vi "Set_Parameter_Instrument (Json).vi"(8 "error in (no error)":errorcluster caption="entrée d'erreur (pas d'erreur)", 10 "Parameter (Json)":string, 11 "Show_Information en entrée":refnum<class "Wait_OpenFixture.lvclass">) -> (0 "error out":errorcluster caption="sortie d'erreur", 3 "Show_Information en sortie":refnum<class "Wait_OpenFixture.lvclass">)   [LabVIEW 2020, in "Library Test.lvlib" / "Wait_OpenFixture.lvclass"]
uses:
  Wait_OpenFixture.lvclass
  C:/Users/ngarcin/OneDrive - Altyor/Standard TB/Class/Test/Test (Default)/Test (Default).lvclass
  Commun VI/TypeDef/Commande DIO/Parameter DIO.ctl
  DIO/Class DIO (Default)/Class DIO (Default).lvclass
  Wait_OpenFixture.lvclass/Wait_OpenFixture.ctl
  JSON API/JSON Value/Set from JSON string.vi
  JSON API/Variant JSON/Variant to JSON.vi
  JSON API/JSON Value/Get Item by name array.vi
  Test_Without_Instr/Test_Without_Inst.lvclass
  Instrument/Instrument (Default)/Class Instrument (Default).lvclass
  JSON API/JSON Value/JSON Value.lvclass
  JSON API/Variant JSON/Variant JSON.lvlib
  JSON API/Get Polymorphic/JSON GetSet.lvlib
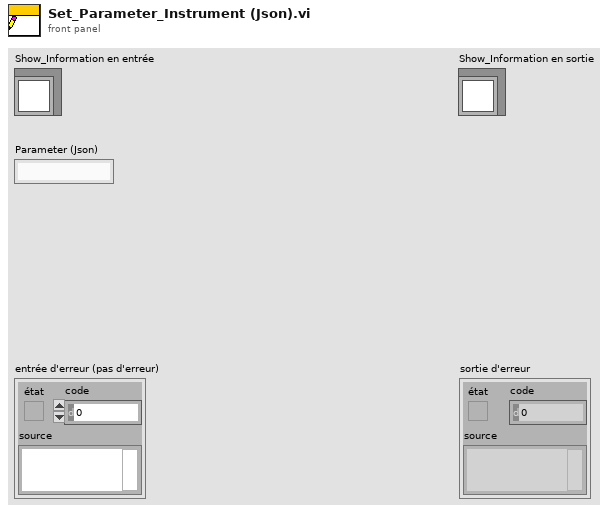
[diagram p1: front panel]
types:
  T1 = cluster{"Information_Operator":string, "Ok_Button_Visible":bool, "Path_Picture":path, "Timeout (ms)":u64, "Function":enum16{"Write", "Read"}, "Line":u8, "Port":u8}
  T2 = typedef "Parameter DIO.ctl" = cluster{"Device_Com_Port":string, "Port":u8, "Line":u8, "Function":enum16{"Write", "Read"}, "Class DIO":refnum<class "Class DIO (Default).lvclass">}
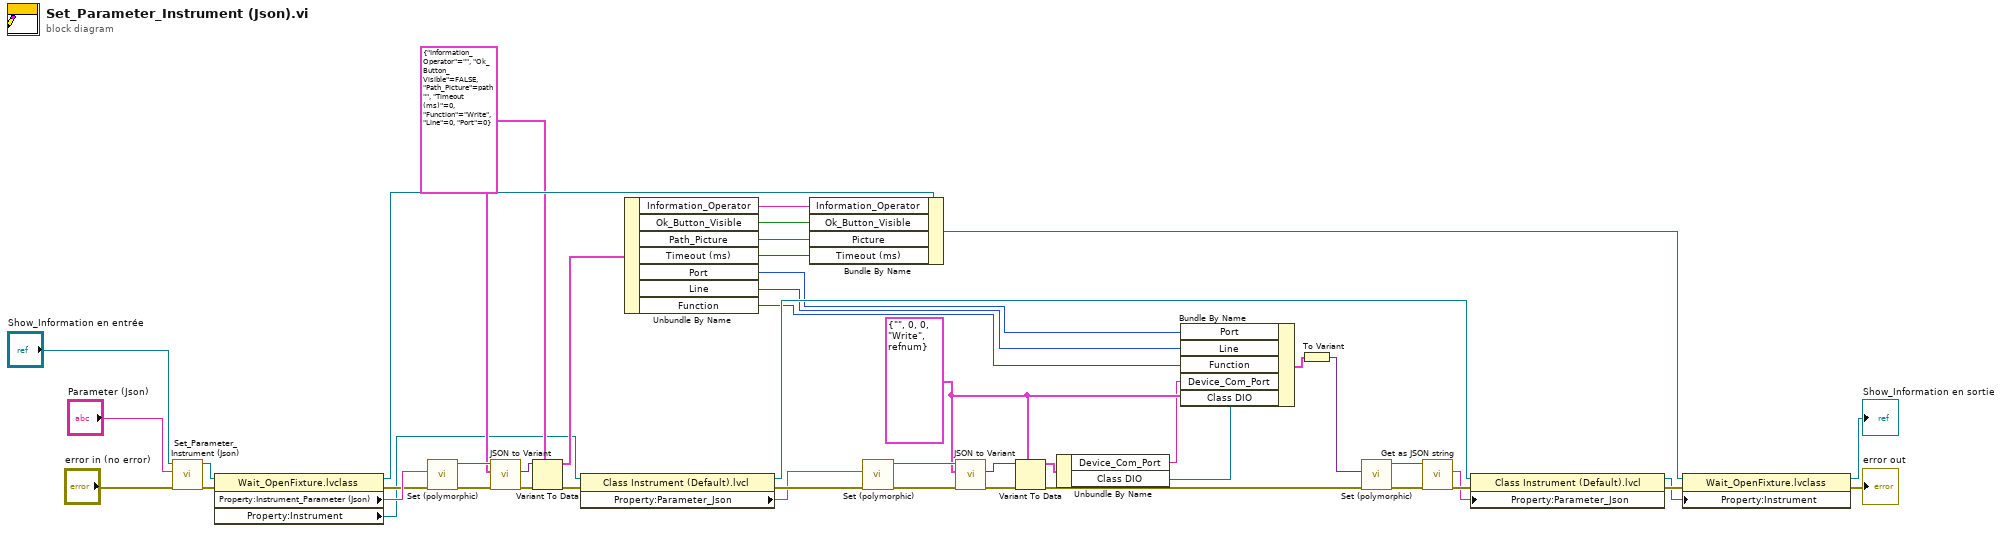
[diagram p0: block diagram]
diagram:
  w12 = T1 {"Information_Operator"="", "Ok_Button_Visible"=FALSE, "Path_Picture"=path "", "Timeout (ms)"=0, "Function"=enum."Write", "Line"=0, "Port"=0} ("Cluster des données privées de classe")
  w19 = T2 {"Device_Com_Port"="", "Port"=0, "Line"=0, "Function"=enum."Write", "Class DIO"=refnum} ("Parameter")
  n1 = call-parent "Set_Parameter_Instrument (Json).vi"("error in (no error)"="error in (no error)", "Parameter (Json)"="Parameter (Json)", "Test (Default) en entrée"="Show_Information en entrée") -> ("error out"=w36:errorcluster, "Test (Default) en sortie"=w37:refnum<class "Wait_OpenFixture.lvclass">)  [unwired: 7 in]
  n2 = property class="Wait_OpenFixture.lvclass"(reference=w37, error in=w36) -> (reference out=w35:refnum<class "Wait_OpenFixture.lvclass">, error out=w42:errorcluster, "Property:Instrument_Parameter (Json)"=w43:string, "Property:Instrument"=w11:refnum<class "Class Instrument (Default).lvclass">)
  n3 = call-poly "Set (polymorphic).vi"("error in (no error)"=w42, "JSON stream"=w43) -> ("error out"=w39:errorcluster, "JSON Value out"=w41:refnum<class "JSON Value.lvclass">)  [unwired: 7 in, 1 out]
  n4 = call "JSON to Variant.vi"("error in (no error)"=w39, "Variant (Data Type)"=w12, "JSON Value"=w41) -> ("error out"=w40:errorcluster, "Variant out"=w38:variant)  [unwired: 7 in]
  n5 = Variant To Data(error in=w40, type=w12, Variant=w38) -> (data=w34:T1, error out=w10:errorcluster)
  n6 = property class="Class Instrument (Default).lvcl"(reference=w11, error in=w10) -> (reference out=w13:refnum<class "Class Instrument (Default).lvclass">, error out=w18:errorcluster, "Property:Parameter_Json"=w14:string)
  n7 = Unbundle By Name(w34) -> ("Information_Operator"=w33:string, "Ok_Button_Visible"=w32:bool, "Path_Picture"=w31:path, "Timeout (ms)"=w30:u64, "Port"=w9:u8, "Line"=w8:u8, "Function"=w7:enum16{"Write", "Read"})
  n8 = Bundle By Name(cluster=w35, "Information_Operator"=w33, "Ok_Button_Visible"=w32, "Picture"=w31, "Timeout (ms)"=w30) -> (w6:refnum<class "Wait_OpenFixture.lvclass">)
  n9 = call-poly "Set (polymorphic).vi"("error in (no error)"=w18, "JSON stream"=w14) -> ("error out"=w22:errorcluster, "JSON Value out"=w20:refnum<class "JSON Value.lvclass">)  [unwired: 7 in, 1 out]
  n10 = call "JSON to Variant.vi"("error in (no error)"=w22, "Variant (Data Type)"=w19, "JSON Value"=w20) -> ("error out"=w21:errorcluster, "Variant out"=w23:variant)  [unwired: 7 in]
  n11 = Variant To Data(error in=w21, type=w19, Variant=w23) -> (data=w16:T2, error out=w17:errorcluster)
  n12 = Unbundle By Name(w16) -> ("Device_Com_Port"=w15:string, "Class DIO"=w1:refnum<class "Class DIO (Default).lvclass">)
  n13 = Bundle By Name(cluster=w19, "Port"=w9, "Line"=w8, "Function"=w7, "Device_Com_Port"=w15, "Class DIO"=w1) -> (w25:T2)
  n14 = To Variant(anything=w25) -> (Variant=w29:variant)
  n15 = call-poly "Set (polymorphic).vi"("error in (no error)"=w17, "Variant"=w29) -> ("error out"=w27:errorcluster, "JSON Value out"=w28:refnum<class "JSON Value.lvclass">)  [unwired: 8 in]
  n16 = call "Get as JSON string.vi"("error in (no error)"=w27, "JSON Value in"=w28) -> ("error out"=w26:errorcluster, "<JSON>"=w24:string)  [unwired: 8 in]
  n17 = property class="Class Instrument (Default).lvcl"(reference=w13, error in=w26, "Property:Parameter_Json"=w24) -> (reference out=w2:refnum<class "Class Instrument (Default).lvclass">, error out=w4:errorcluster)
  n18 = property class="Wait_OpenFixture.lvclass"(reference=w6, error in=w4, "Property:Instrument"=w2) -> (reference out=→"Show_Information en sortie":refnum<class "Wait_OpenFixture.lvclass">, error out=→"error out":errorcluster)
